vi "GetExampleImage.vi"(8 "error in":errorcluster, 11 "File Path":path) -> (0 "error out":errorcluster, 3 "path":path)   [LabVIEW 2020, in "OpenLvVision_Overlays.lvlib"]
doc: "Thirdparty:\n© 2000–2025 National Instruments Corporation. All rights reserved.\n\nThird party copyrights are property of their respective owners."
uses:
  OpenLvVision_Overlays.lvlib
  <vilib>/registry/registry.llb/Registry SAM.ctl
  <vilib>/registry/registry.llb/Read Registry Value Simple STR.vi
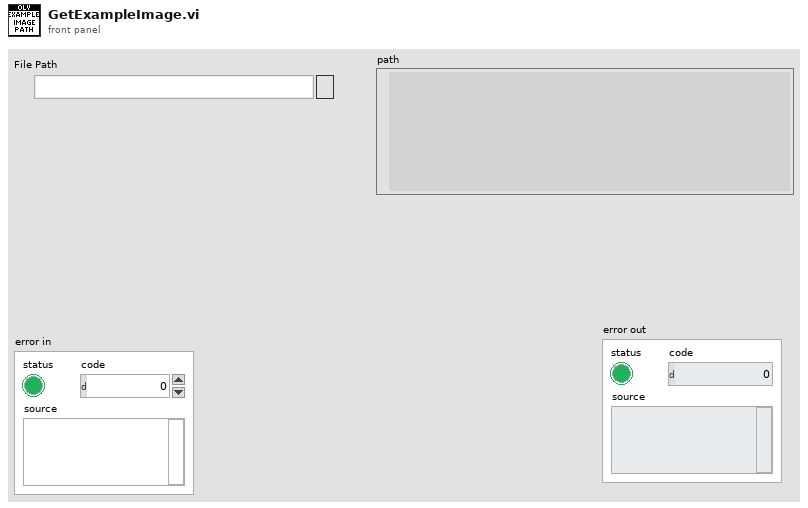
[diagram p1: front panel]
types:
  T1 = typedef "Registry SAM.ctl" = enum32{"KEY_QUERY_VALUE", "KEY_SET_VALUE", "KEY_CREATE_SUB_KEY", "KEY_ENUMERATE_SUB_KEYS", "KEY_NOTIFY", "KEY_CREATE_LINK", "KEY_READ", "KEY_WRITE", "KEY_ALL_ACCESS", "KEY_READ | KEY_WRITE"}
  T2 = typedef "Registry refnum.ctl" = refnum<k1>
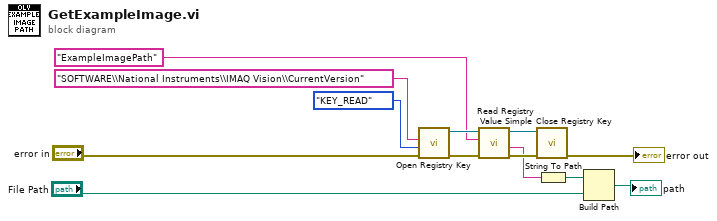
[diagram p0: block diagram]
diagram:
  n1 = call <vilib>:"Open Registry Key.vi"("error in (no error)"="error in", "security access mask (KEY_READ | KEY_WRITE)"=Registry_SAM."KEY_READ", "subkey"="SOFTWARE\\National Instruments\\IMAQ Vision\\CurrentVersion") -> ("error out"=w12:errorcluster, "refnum out"=w11:T2)  [unwired: 7 in]
  n2 = call-poly <vilib>:"Read Registry Value Simple.vi"("error in (no error)"=w12, "value"="ExampleImagePath", "refnum"=w11) -> ("error out"=w9:errorcluster, "String/Binary data"=w7:string, "refnum out"=w8:T2)  [unwired: 3 in, 1 out]
  n3 = call <vilib>:"Close Registry Key.vi"("error in (no error)"=w9, "refnum"=w8) -> ("error out"=→"error out":errorcluster)  [unwired: 5 in]
  n4 = String To Path(string=w7) -> (path=w5:path)
  n5 = Build Path(base path=w5, name or relative path="File Path") -> (appended path=→"path":path)
